vi "HS_ReadTxBuffer.vi"(8 "error in":errorcluster, 9 "Console In":string, 11 "VISA Refnum in":refnum<visa-resource-name>) -> (0 "error out":errorcluster, 1 "Console Out":string, 2 "Tx Buffer":string, 3 "VISA Refnum out":refnum<visa-resource-name>)   [LabVIEW 2016]
panel:
  out "tx_len":u32
  out "Tx Buffer Len":string
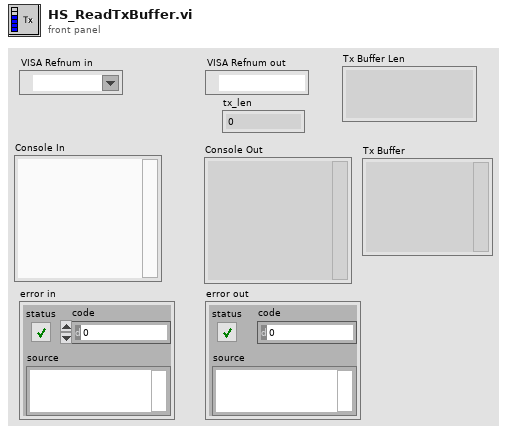
[diagram p1: front panel]
types:
  T1 = cluster{"Before":u8, "After":u8, "Send as 1 block?":bool}
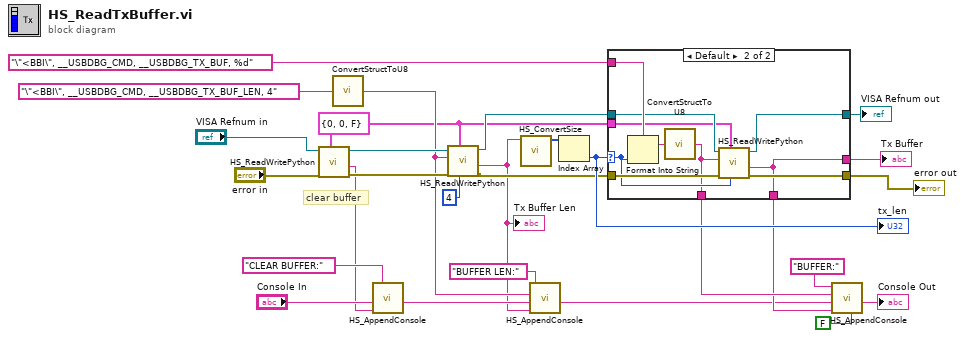
[diagram p0: block diagram]
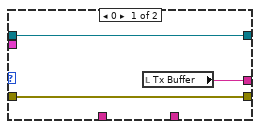
[diagram p2: hidden frame]
diagram:
  w3 = T1 {"Before"=0, "After"=0, "Send as 1 block?"=FALSE} ("Timeouts (ms)")
  # "clear buffer"
  n1 = call "HS_ReadWritePython.vi"("Timeouts (ms)"=w3, "error in"="error in", "VISA in"="VISA Refnum in") -> ("error out"=w17:errorcluster, "Console Out"=w14:string, "VISA out"=w19:refnum<visa-resource-name>)  [unwired: 3 in, 3 out]
  n2 = call "ConvertStructToU8.vi"("struct"="\"<BBI\", __USBDBG_CMD, __USBDBG_TX_BUF_LEN, 4" ("write buffer")) -> ("Binary"=w4:string)
  n3 = call "HS_AppendConsole.vi"("Reply"=w14, "Console in"="Console In", "Command"="CLEAR BUFFER:") -> ("Console Out"=w12:string)  [unwired: 8 in]
  n4 = call "HS_ReadWritePython.vi"("Reply length"=4, "Timeouts (ms)"=w3, "error in"=w17, "Write"=w4, "VISA in"=w19) -> ("error out"=w23:errorcluster, "Console Out"=w1:string, "VISA out"=w22:refnum<visa-resource-name>)  [unwired: 1 in, 3 out]
  "Tx Buffer Len" <- w1
  n5 = call "HS_ConvertSize.vi"("read buffer"=w1) -> ("size()"=w21:u32[])  [unwired: 9 in, 1 out]
  n6 = call "HS_AppendConsole.vi"("Reply"=w1, "Console in"=w12, "Send"=w4, "Command"="BUFFER LEN:") -> ("Console Out"=w8:string)  [unwired: 7 in]
  n7 = Index Array(array=w21) -> (element=w28:u32)  [unwired: 1 in]
  "tx_len" <- w28
  n8 = case shown="Default" w28 {
    selector: w28 -> [_ w36]
    tunnel: w22 -> [w31 w39]
    tunnel: w23 -> [w30 w38]
    tunnel: [w30 w37] -> w25
    tunnel: [w31 w35] -> w26
    tunnel: "\"<BBI\", __USBDBG_CMD, __USBDBG_TX_BUF, %d" ("write buffer") -> [_ w41]
    tunnel: [w29 w33] -> w20
    tunnel: [_ w34] -> w10
    tunnel: [_ w33] -> w9
    tunnel: w3 -> [_ w32]
    frame 0 {
      n9 = local read "Tx Buffer"() -> (w29:string)
    }
    frame Default {
      n10 = Format Into String(format string=w41, w36) -> (resulting string=w40:string)  [unwired: 2 in, 1 out]
      n11 = call "ConvertStructToU8.vi"("struct"=w40) -> ("Binary"=w34:string)
      n12 = call "HS_ReadWritePython.vi"("Reply length"=w36, "Timeouts (ms)"=w32, "error in"=w38, "Write"=w34, "VISA in"=w39) -> ("error out"=w37:errorcluster, "Console Out"=w33:string, "VISA out"=w35:refnum<visa-resource-name>)  [unwired: 1 in, 3 out]
    }
  }
  "Tx Buffer" <- w20
  "VISA Refnum out" <- w26
  "error out" <- w25
  n13 = call "HS_AppendConsole.vi"("Show Reply Binary?"=FALSE, "Reply"=w9, "Console in"=w8, "Send"=w10, "Command"="BUFFER:") -> ("Console Out"=→"Console Out":string)  [unwired: 6 in]
